vi "DelayTimeCorrection.vi"(0 "ReS":dbl, 5 "ImS":dbl, 7 "Frequency":dbl, 9 "Dealy Time":dbl, 11 "error in (no error)":errorcluster) -> (4 "ReS_corrected":dbl, 6 "ImS_corrected":dbl, 15 "error out":errorcluster)   [LabVIEW 2015]
uses:
  <vilib>/express/express arith-compare/Formula/XNode/ExpressFormulaBlockNode.xnode
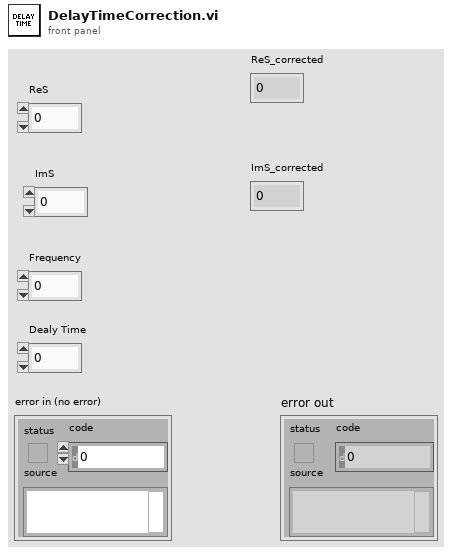
[diagram p1: front panel]
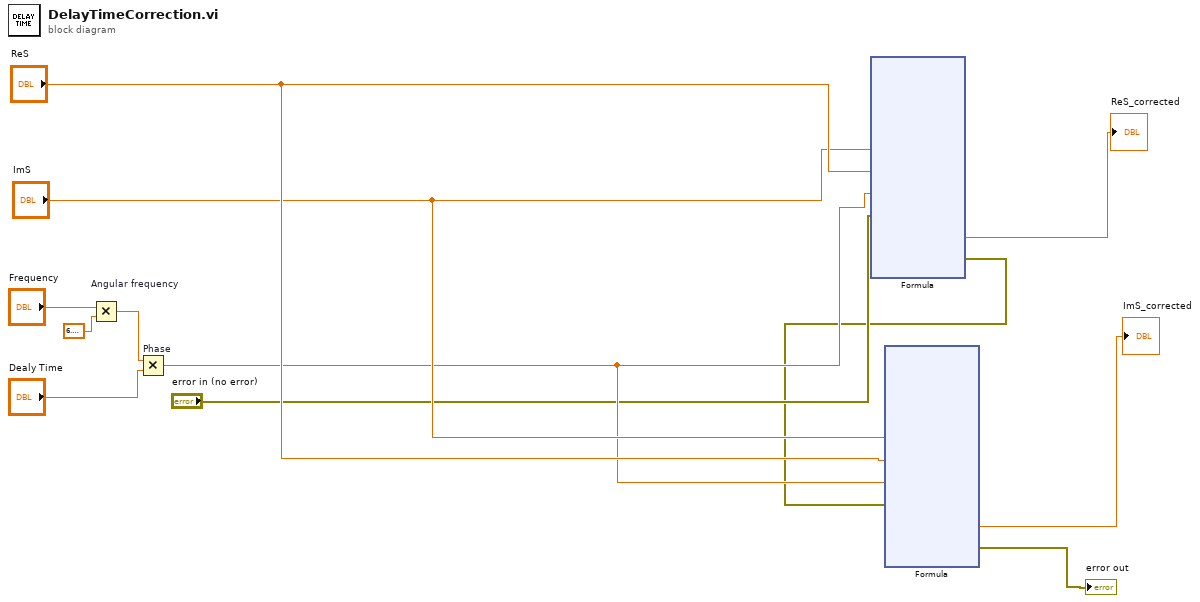
[diagram p0: block diagram]
diagram:
  n1 = Multiply "Angular frequency"(x="Frequency", y=6.283185307179586) -> (x*y=w9:dbl)
  n2 = Multiply "Phase"(x=w9, y="Dealy Time") -> (x*y=w4:dbl)
  n3 = xnode "Formula"("ImS"="ImS", "ReS"="ReS", "phase"=w4, "error in (no error)"="error in (no error)") -> ("Result"=→"ReS_corrected":dbl, "error out"=w2:errorcluster)
  n4 = xnode "Formula"("ImS"="ImS", "ReS"="ReS", "phase"=w4, "error in (no error)"=w2) -> ("Result"=→"ImS_corrected":dbl, "error out"=→"error out":errorcluster)
